vi "Read Script from File and Write to HSDIO.vi"(7 "Script_Name":string, 8 "Error In":errorcluster, 11 "Semiconductor Module Context":T1) -> (0 "Error Out":errorcluster)   [LabVIEW 2013]
uses:
  <vilib>/NI_TestStand_SemiconductorModule/NI_TestStand_Semiconductor_Module.lvlibp/PinMap/General/SemiconductorModuleContext.ctl
  <vilib>/NI_TestStand_SemiconductorModule/NI_TestStand_Semiconductor_Module.lvlibp
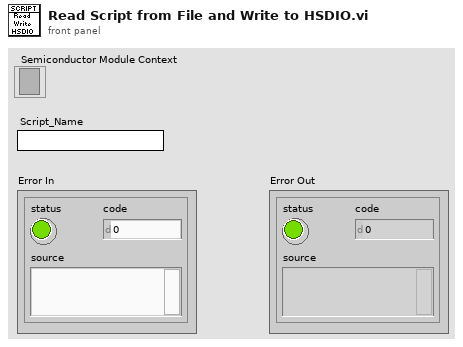
[diagram p1: front panel]
types:
  T1 = typedef "NI_TestStand_Semiconductor_Module.lvlibp/SemiconductorModuleContext.ctl" = refnum<k7>
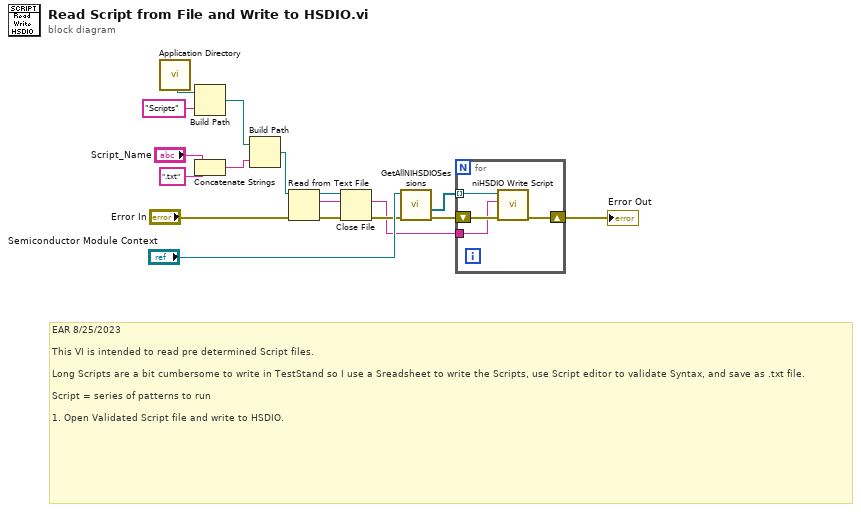
[diagram p0: block diagram]
diagram:
  # "EAR 8/25/2023\n\nThis VI is intended to read pre determined Script files. \n\nLong Scripts are a bit cumbersome to write in TestStand so I use a Sreadsheet to write the Scripts, use Script editor to validate Syntax, and save as .txt file.\n\nScript = series of patterns to run\n\n1. Open Validated Script file and write to HSDIO."
  n1 = call <vilib>:"Application Directory.vi"() -> ("Application Directory"=w13:path)
  n2 = Build Path(base path=w13, name or relative path="Scripts") -> (appended path=w11:path)
  n3 = Concatenate Strings("Script_Name", ".txt" ("string")) -> (w8:string)
  n4 = Build Path(base path=w11, name or relative path=w8) -> (appended path=w7:path)
  n5 = Read from Text File(file (use dialog)=w7, error in="Error In") -> (refnum out=w4:refnum<file>, text=w2:string, error out=w5:errorcluster)  [unwired: 2 in, 1 out]
  n6 = Close File(refnum=w4, error in=w5) -> (error out=w3:errorcluster)  [unwired: 1 out]
  n7 = call <vilib>:"GetAllNIHSDIOSessions.vi"("error in (no error)"=w3, "Semiconductor Module Context"="Semiconductor Module Context") -> ("error out"=w16:errorcluster, "Generation Sessions"=w15:refnum<k15>[])  [unwired: 6 in, 2 out]
  n8 = for {
    tunnel: w15 -> [w19] mode=indexing
    shift-right: [w18] -> w1
    shift-left: w16 -> [w20]
    tunnel: w2 -> [w17]
    n9 = call <instrlib>:"niHSDIO Write Script.vi"("error in (no error)"=w20, "script"=w17, "instrument handle"=w19) -> ("error out"=w18:errorcluster)  [unwired: 7 in, 1 out]
  }
  "Error Out" <- w1
